vi "calcular_temp_ntc.vi"(1 "Vin":dbl) -> (0 "temp_ntc":dbl)   [LabVIEW 2018]
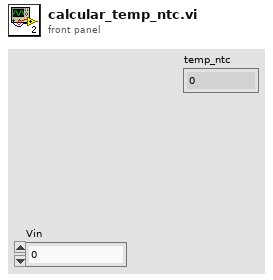
[diagram p1: front panel]
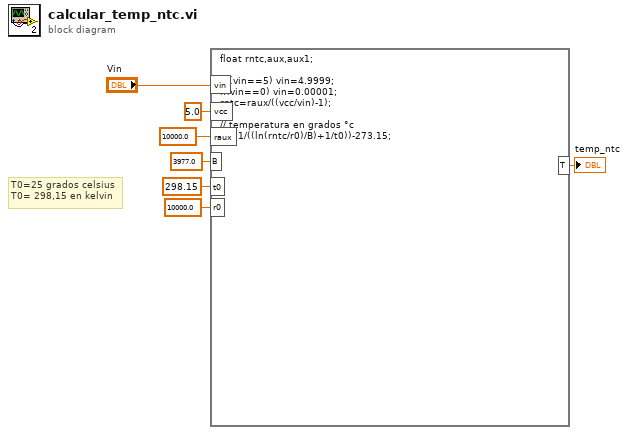
[diagram p0: block diagram]
diagram:
  # "T0=25 grados celsius\nT0= 298,15 en kelvin"
  n1 = formula code="float rntc,aux,aux1;\n\nif (vin==5) vin=4.9999;\nif(vin==0) vin=0.00001;\nrntc=raux/((vcc/vin)-1);\n\n// temperatura en grados °c\nT=(1/((ln(rntc/r0)/B)+1/t0))-273.15;"("vin"="Vin", "vcc"=5.0 ("input variable"), "raux"=10000.0 ("input variable"), "B"=3977.0 ("input variable"), "t0"=298.15 ("input variable"), "r0"=10000.0 ("input variable")) -> ("T"=→"temp_ntc":dbl)
